vi "rs3 set filter options.vi"(8 "error in (no error)":errorcluster, 10 "Processing Blocks":T2, 11 "Filter settings":T1={"Decimation Scale (1-10)"=3, "Spatial Alpha (0-1)"=0.6, "Spatial Delta (1/32 disp)"=8, "Temporal Alpha (0-1)"=0.4, "Temporal Delta (1/32 disp)"=20, "Persistence (0= none, 8=max)"=0, "spatial holefill radius (0 disable, 5 max) "=0, "spatial iteration (2=default)"=2} {"spatial iteration (2=default)" min=1 max=10; "Decimation Scale (1-10)" min=1 max=10; "Spatial Alpha (0-1)" min=0 max=1 format="%_2g"; "Spatial Delta (1/32 disp)" min=1; "Temporal Alpha (0-1)" min=0 max=1 format="%_2g"; "Temporal Delta (1/32 disp)" min=1; "Persistence (0= none, 8=max)" max=8; "spatial holefill radius (0 disable, 5 max)" max=5}) -> (0 "error out":errorcluster)   [LabVIEW 2017, in "libRealSense3.lvlib"]
doc: "Sets post-processing filter options."
uses:
  libRealSense3.lvlib
panel:
  # "RS3 Set Filter Options"
  # "Spatial Holefill:       \n        0= disabled,\n        1= 2_pixel_radius,\n        2= 4_pixel_radius,\n        3= 8_pixel_radius,\n        4= 6_pixel_radius,\n        5= unlimited_radius"
  # "(C) Intel Corp.,  AGJ"
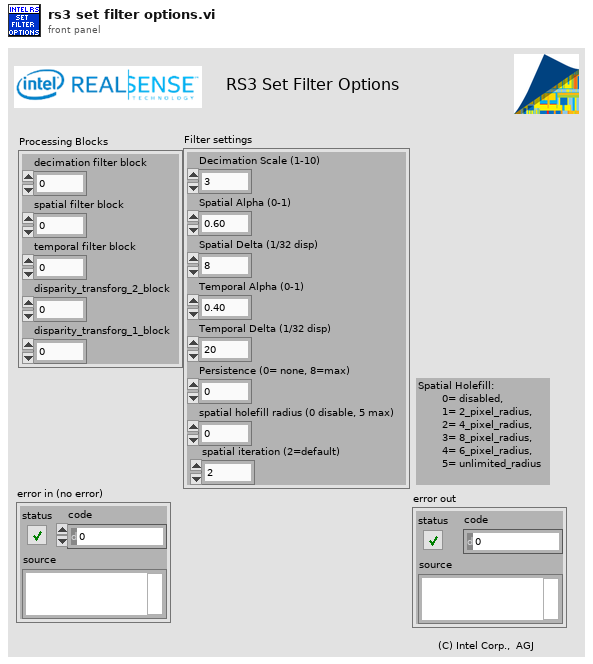
[diagram p1: front panel]
types:
  T1 = cluster{"Decimation Scale (1-10)":u8, "Spatial Alpha (0-1)":sgl, "Spatial Delta (1/32 disp)":u16, "Temporal Alpha (0-1)":sgl, "Temporal Delta (1/32 disp)":u16, "Persistence (0= none, 8=max)":u8, "spatial holefill radius (0 disable, 5 max) ":u8, "spatial iteration (2=default)":u8}
  T2 = cluster{"decimation filter block":u64, "spatial filter block":u64, "temporal filter block":u64, "disparity_transforg_2_block":u64, "disparity_transforg_1_block":u64}
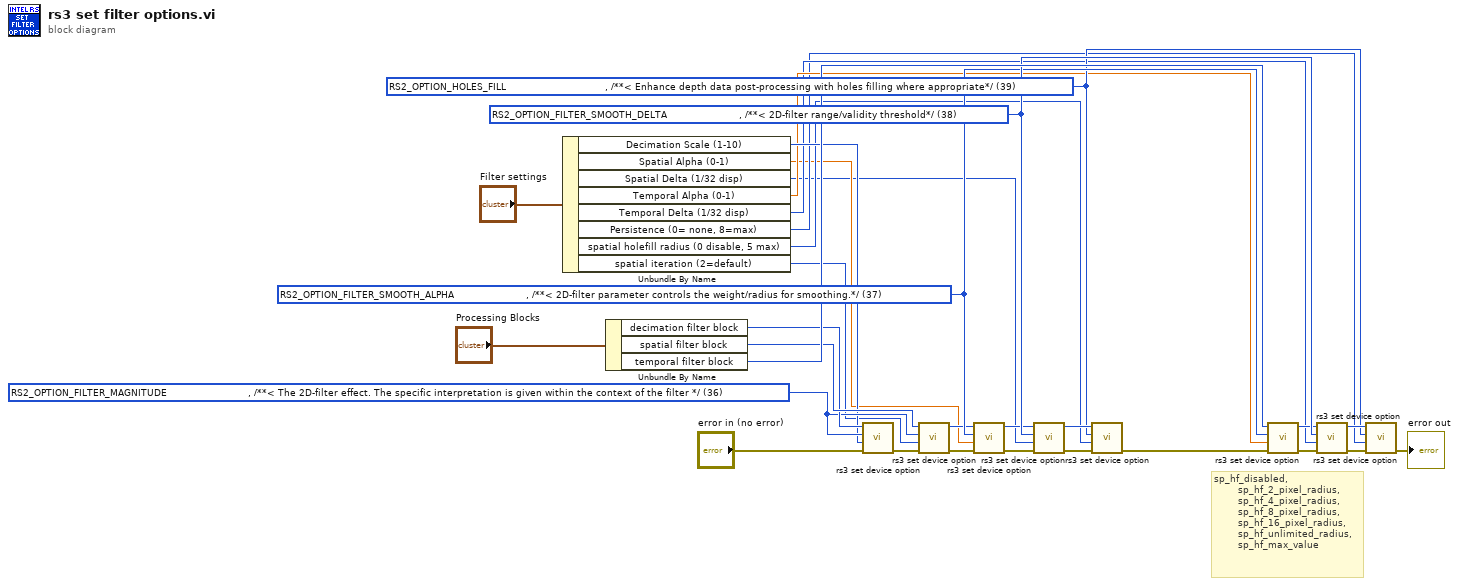
[diagram p0: block diagram]
diagram:
  w9 = u16 39 items=["    RS2_OPTION_BACKLIGHT_COMPENSATION                     , /**< Enable / disable color backlight compensation*/", "    RS2_OPTION_BRIGHTNESS                                 , /**< Color image brightness*/", "    RS2_OPTION_CONTRAST                                   , /**< Color image contrast*/", "    RS2_OPTION_EXPOSURE                                   , /**< Controls exposure time of color camera. Setting any value will disable auto exposure*/", "    RS2_OPTION_GAIN                                       , /**< Color image gain*/", "    RS2_OPTION_GAMMA                                      , /**< Color image gamma setting*/", "    RS2_OPTION_HUE                                        , /**< Color image hue*/", "    RS2_OPTION_SATURATION                                 , /**< Color image saturation setting*/", "    RS2_OPTION_SHARPNESS                                  , /**< Color image sharpness setting*/", "    RS2_OPTION_WHITE_BALANCE                              , /**< Controls white balance of color image. Setting any value will disable auto white balance*/", "    RS2_OPTION_ENABLE_AUTO_EXPOSURE                       , /**< Enable / disable color image auto-exposure*/", "    RS2_OPTION_ENABLE_AUTO_WHITE_BALANCE                  , /**< Enable / disable color image auto-white-balance*/", "    RS2_OPTION_VISUAL_PRESET                              , /**< Provide access to several recommend sets of option presets for the depth camera */", "    RS2_OPTION_LASER_POWER                                , /**< Power of the F200 / SR300 projector, with 0 meaning projector off*/", "    RS2_OPTION_ACCURACY                                   , /**< Set the number of patterns projected per frame. The higher the accuracy value the more patterns projected. Increasing the number of patterns help to achieve better accuracy. Note that this c", "    RS2_OPTION_MOTION_RANGE                               , /**< Motion vs. Range trade-off, with lower values allowing for better motion sensitivity and higher values allowing for better depth range*/", "    RS2_OPTION_FILTER_OPTION                              , /**< Set the filter to apply to each depth frame. Each one of the filter is optimized per the application requirements*/", "    RS2_OPTION_CONFIDENCE_THRESHOLD                       , /**< The confidence level threshold used by the Depth algorithm pipe to set whether a pixel will get a valid range or will be marked with invalid range*/", "    RS2_OPTION_EMITTER_ENABLED                            , /**< Laser Emitter enabled */", "    RS2_OPTION_FRAMES_QUEUE_SIZE                          , /**< Number of frames the user is allowed to keep per stream. Trying to hold-on to more frames will cause frame-drops.*/", "    RS2_OPTION_TOTAL_FRAME_DROPS                          , /**< Total number of detected frame drops from all streams */", "    RS2_OPTION_AUTO_EXPOSURE_MODE                         , /**< Auto-Exposure modes: Static, Anti-Flicker and Hybrid */", "    RS2_OPTION_POWER_LINE_FREQUENCY                       , /**< Power Line Frequency control for anti-flickering Off/50Hz/60Hz/Auto */", "    RS2_OPTION_ASIC_TEMPERATURE                           , /**< Current Asic Temperature */", "    RS2_OPTION_ERROR_POLLING_ENABLED                      , /**< disable error handling */", "    RS2_OPTION_PROJECTOR_TEMPERATURE                      , /**< Current Projector Temperature */", "    RS2_OPTION_OUTPUT_TRIGGER_ENABLED                     , /**< Enable / disable trigger to be outputed from the camera to any external device on every depth frame */", "    RS2_OPTION_MOTION_MODULE_TEMPERATURE                  , /**< Current Motion-Module Temperature */", "    RS2_OPTION_DEPTH_UNITS                                , /**< Number of meters represented by a single depth unit */", "    RS2_OPTION_ENABLE_MOTION_CORRECTION                   , /**< Enable/Disable automatic correction of the motion data */", "    RS2_OPTION_AUTO_EXPOSURE_PRIORITY                     , /**< Allows sensor to dynamically ajust the frame rate depending on lighting conditions */", "    RS2_OPTION_COLOR_SCHEME                               , /**< Color scheme for data visualization */", "    RS2_OPTION_HISTOGRAM_EQUALIZATION_ENABLED             , /**< Perform histogram equalization post-processing on the depth data */", "    RS2_OPTION_MIN_DISTANCE                               , /**< Minimal distance to the target */", "    RS2_OPTION_MAX_DISTANCE                               , /**< Maximum distance to the target */", "    RS2_OPTION_TEXTURE_SOURCE                             , /**< Texture mapping stream unique ID */", "    RS2_OPTION_FILTER_MAGNITUDE                           , /**< The 2D-filter effect. The specific interpretation is given within the context of the filter */", "    RS2_OPTION_FILTER_SMOOTH_ALPHA                        , /**< 2D-filter parameter controls the weight/radius for smoothing.*/", "    RS2_OPTION_FILTER_SMOOTH_DELTA                        , /**< 2D-filter range/validity threshold*/", "    RS2_OPTION_HOLES_FILL                                 , /**< Enhance depth data post-processing with holes filling where appropriate*/", "    RS2_OPTION_STEREO_BASELINE                            , /**< The distance in mm between the first and the second imagers in stereo-based depth cameras*/", "    RS2_OPTION_AUTO_EXPOSURE_CONVERGE_STEP                , /**< Allows dynamically ajust the converge step value of the target exposure in Auto-Exposure algorithm*/", "    RS2_OPTION_COUNT                                        /**< Number of enumeration values. Not a valid input: intended to be used in for-loops. */"] ("RS Option")
  w24 = u16 38 items=["    RS2_OPTION_BACKLIGHT_COMPENSATION                     , /**< Enable / disable color backlight compensation*/", "    RS2_OPTION_BRIGHTNESS                                 , /**< Color image brightness*/", "    RS2_OPTION_CONTRAST                                   , /**< Color image contrast*/", "    RS2_OPTION_EXPOSURE                                   , /**< Controls exposure time of color camera. Setting any value will disable auto exposure*/", "    RS2_OPTION_GAIN                                       , /**< Color image gain*/", "    RS2_OPTION_GAMMA                                      , /**< Color image gamma setting*/", "    RS2_OPTION_HUE                                        , /**< Color image hue*/", "    RS2_OPTION_SATURATION                                 , /**< Color image saturation setting*/", "    RS2_OPTION_SHARPNESS                                  , /**< Color image sharpness setting*/", "    RS2_OPTION_WHITE_BALANCE                              , /**< Controls white balance of color image. Setting any value will disable auto white balance*/", "    RS2_OPTION_ENABLE_AUTO_EXPOSURE                       , /**< Enable / disable color image auto-exposure*/", "    RS2_OPTION_ENABLE_AUTO_WHITE_BALANCE                  , /**< Enable / disable color image auto-white-balance*/", "    RS2_OPTION_VISUAL_PRESET                              , /**< Provide access to several recommend sets of option presets for the depth camera */", "    RS2_OPTION_LASER_POWER                                , /**< Power of the F200 / SR300 projector, with 0 meaning projector off*/", "    RS2_OPTION_ACCURACY                                   , /**< Set the number of patterns projected per frame. The higher the accuracy value the more patterns projected. Increasing the number of patterns help to achieve better accuracy. Note that this c", "    RS2_OPTION_MOTION_RANGE                               , /**< Motion vs. Range trade-off, with lower values allowing for better motion sensitivity and higher values allowing for better depth range*/", "    RS2_OPTION_FILTER_OPTION                              , /**< Set the filter to apply to each depth frame. Each one of the filter is optimized per the application requirements*/", "    RS2_OPTION_CONFIDENCE_THRESHOLD                       , /**< The confidence level threshold used by the Depth algorithm pipe to set whether a pixel will get a valid range or will be marked with invalid range*/", "    RS2_OPTION_EMITTER_ENABLED                            , /**< Laser Emitter enabled */", "    RS2_OPTION_FRAMES_QUEUE_SIZE                          , /**< Number of frames the user is allowed to keep per stream. Trying to hold-on to more frames will cause frame-drops.*/", "    RS2_OPTION_TOTAL_FRAME_DROPS                          , /**< Total number of detected frame drops from all streams */", "    RS2_OPTION_AUTO_EXPOSURE_MODE                         , /**< Auto-Exposure modes: Static, Anti-Flicker and Hybrid */", "    RS2_OPTION_POWER_LINE_FREQUENCY                       , /**< Power Line Frequency control for anti-flickering Off/50Hz/60Hz/Auto */", "    RS2_OPTION_ASIC_TEMPERATURE                           , /**< Current Asic Temperature */", "    RS2_OPTION_ERROR_POLLING_ENABLED                      , /**< disable error handling */", "    RS2_OPTION_PROJECTOR_TEMPERATURE                      , /**< Current Projector Temperature */", "    RS2_OPTION_OUTPUT_TRIGGER_ENABLED                     , /**< Enable / disable trigger to be outputed from the camera to any external device on every depth frame */", "    RS2_OPTION_MOTION_MODULE_TEMPERATURE                  , /**< Current Motion-Module Temperature */", "    RS2_OPTION_DEPTH_UNITS                                , /**< Number of meters represented by a single depth unit */", "    RS2_OPTION_ENABLE_MOTION_CORRECTION                   , /**< Enable/Disable automatic correction of the motion data */", "    RS2_OPTION_AUTO_EXPOSURE_PRIORITY                     , /**< Allows sensor to dynamically ajust the frame rate depending on lighting conditions */", "    RS2_OPTION_COLOR_SCHEME                               , /**< Color scheme for data visualization */", "    RS2_OPTION_HISTOGRAM_EQUALIZATION_ENABLED             , /**< Perform histogram equalization post-processing on the depth data */", "    RS2_OPTION_MIN_DISTANCE                               , /**< Minimal distance to the target */", "    RS2_OPTION_MAX_DISTANCE                               , /**< Maximum distance to the target */", "    RS2_OPTION_TEXTURE_SOURCE                             , /**< Texture mapping stream unique ID */", "    RS2_OPTION_FILTER_MAGNITUDE                           , /**< The 2D-filter effect. The specific interpretation is given within the context of the filter */", "    RS2_OPTION_FILTER_SMOOTH_ALPHA                        , /**< 2D-filter parameter controls the weight/radius for smoothing.*/", "    RS2_OPTION_FILTER_SMOOTH_DELTA                        , /**< 2D-filter range/validity threshold*/", "    RS2_OPTION_HOLES_FILL                                 , /**< Enhance depth data post-processing with holes filling where appropriate*/", "    RS2_OPTION_STEREO_BASELINE                            , /**< The distance in mm between the first and the second imagers in stereo-based depth cameras*/", "    RS2_OPTION_AUTO_EXPOSURE_CONVERGE_STEP                , /**< Allows dynamically ajust the converge step value of the target exposure in Auto-Exposure algorithm*/", "    RS2_OPTION_COUNT                                        /**< Number of enumeration values. Not a valid input: intended to be used in for-loops. */"] ("RS Option")
  w23 = u16 37 items=["    RS2_OPTION_BACKLIGHT_COMPENSATION                     , /**< Enable / disable color backlight compensation*/", "    RS2_OPTION_BRIGHTNESS                                 , /**< Color image brightness*/", "    RS2_OPTION_CONTRAST                                   , /**< Color image contrast*/", "    RS2_OPTION_EXPOSURE                                   , /**< Controls exposure time of color camera. Setting any value will disable auto exposure*/", "    RS2_OPTION_GAIN                                       , /**< Color image gain*/", "    RS2_OPTION_GAMMA                                      , /**< Color image gamma setting*/", "    RS2_OPTION_HUE                                        , /**< Color image hue*/", "    RS2_OPTION_SATURATION                                 , /**< Color image saturation setting*/", "    RS2_OPTION_SHARPNESS                                  , /**< Color image sharpness setting*/", "    RS2_OPTION_WHITE_BALANCE                              , /**< Controls white balance of color image. Setting any value will disable auto white balance*/", "    RS2_OPTION_ENABLE_AUTO_EXPOSURE                       , /**< Enable / disable color image auto-exposure*/", "    RS2_OPTION_ENABLE_AUTO_WHITE_BALANCE                  , /**< Enable / disable color image auto-white-balance*/", "    RS2_OPTION_VISUAL_PRESET                              , /**< Provide access to several recommend sets of option presets for the depth camera */", "    RS2_OPTION_LASER_POWER                                , /**< Power of the F200 / SR300 projector, with 0 meaning projector off*/", "    RS2_OPTION_ACCURACY                                   , /**< Set the number of patterns projected per frame. The higher the accuracy value the more patterns projected. Increasing the number of patterns help to achieve better accuracy. Note that this c", "    RS2_OPTION_MOTION_RANGE                               , /**< Motion vs. Range trade-off, with lower values allowing for better motion sensitivity and higher values allowing for better depth range*/", "    RS2_OPTION_FILTER_OPTION                              , /**< Set the filter to apply to each depth frame. Each one of the filter is optimized per the application requirements*/", "    RS2_OPTION_CONFIDENCE_THRESHOLD                       , /**< The confidence level threshold used by the Depth algorithm pipe to set whether a pixel will get a valid range or will be marked with invalid range*/", "    RS2_OPTION_EMITTER_ENABLED                            , /**< Laser Emitter enabled */", "    RS2_OPTION_FRAMES_QUEUE_SIZE                          , /**< Number of frames the user is allowed to keep per stream. Trying to hold-on to more frames will cause frame-drops.*/", "    RS2_OPTION_TOTAL_FRAME_DROPS                          , /**< Total number of detected frame drops from all streams */", "    RS2_OPTION_AUTO_EXPOSURE_MODE                         , /**< Auto-Exposure modes: Static, Anti-Flicker and Hybrid */", "    RS2_OPTION_POWER_LINE_FREQUENCY                       , /**< Power Line Frequency control for anti-flickering Off/50Hz/60Hz/Auto */", "    RS2_OPTION_ASIC_TEMPERATURE                           , /**< Current Asic Temperature */", "    RS2_OPTION_ERROR_POLLING_ENABLED                      , /**< disable error handling */", "    RS2_OPTION_PROJECTOR_TEMPERATURE                      , /**< Current Projector Temperature */", "    RS2_OPTION_OUTPUT_TRIGGER_ENABLED                     , /**< Enable / disable trigger to be outputed from the camera to any external device on every depth frame */", "    RS2_OPTION_MOTION_MODULE_TEMPERATURE                  , /**< Current Motion-Module Temperature */", "    RS2_OPTION_DEPTH_UNITS                                , /**< Number of meters represented by a single depth unit */", "    RS2_OPTION_ENABLE_MOTION_CORRECTION                   , /**< Enable/Disable automatic correction of the motion data */", "    RS2_OPTION_AUTO_EXPOSURE_PRIORITY                     , /**< Allows sensor to dynamically ajust the frame rate depending on lighting conditions */", "    RS2_OPTION_COLOR_SCHEME                               , /**< Color scheme for data visualization */", "    RS2_OPTION_HISTOGRAM_EQUALIZATION_ENABLED             , /**< Perform histogram equalization post-processing on the depth data */", "    RS2_OPTION_MIN_DISTANCE                               , /**< Minimal distance to the target */", "    RS2_OPTION_MAX_DISTANCE                               , /**< Maximum distance to the target */", "    RS2_OPTION_TEXTURE_SOURCE                             , /**< Texture mapping stream unique ID */", "    RS2_OPTION_FILTER_MAGNITUDE                           , /**< The 2D-filter effect. The specific interpretation is given within the context of the filter */", "    RS2_OPTION_FILTER_SMOOTH_ALPHA                        , /**< 2D-filter parameter controls the weight/radius for smoothing.*/", "    RS2_OPTION_FILTER_SMOOTH_DELTA                        , /**< 2D-filter range/validity threshold*/", "    RS2_OPTION_HOLES_FILL                                 , /**< Enhance depth data post-processing with holes filling where appropriate*/", "    RS2_OPTION_STEREO_BASELINE                            , /**< The distance in mm between the first and the second imagers in stereo-based depth cameras*/", "    RS2_OPTION_AUTO_EXPOSURE_CONVERGE_STEP                , /**< Allows dynamically ajust the converge step value of the target exposure in Auto-Exposure algorithm*/", "    RS2_OPTION_COUNT                                        /**< Number of enumeration values. Not a valid input: intended to be used in for-loops. */"] ("RS Option")
  w16 = u16 36 items=["    RS2_OPTION_BACKLIGHT_COMPENSATION                     , /**< Enable / disable color backlight compensation*/", "    RS2_OPTION_BRIGHTNESS                                 , /**< Color image brightness*/", "    RS2_OPTION_CONTRAST                                   , /**< Color image contrast*/", "    RS2_OPTION_EXPOSURE                                   , /**< Controls exposure time of color camera. Setting any value will disable auto exposure*/", "    RS2_OPTION_GAIN                                       , /**< Color image gain*/", "    RS2_OPTION_GAMMA                                      , /**< Color image gamma setting*/", "    RS2_OPTION_HUE                                        , /**< Color image hue*/", "    RS2_OPTION_SATURATION                                 , /**< Color image saturation setting*/", "    RS2_OPTION_SHARPNESS                                  , /**< Color image sharpness setting*/", "    RS2_OPTION_WHITE_BALANCE                              , /**< Controls white balance of color image. Setting any value will disable auto white balance*/", "    RS2_OPTION_ENABLE_AUTO_EXPOSURE                       , /**< Enable / disable color image auto-exposure*/", "    RS2_OPTION_ENABLE_AUTO_WHITE_BALANCE                  , /**< Enable / disable color image auto-white-balance*/", "    RS2_OPTION_VISUAL_PRESET                              , /**< Provide access to several recommend sets of option presets for the depth camera */", "    RS2_OPTION_LASER_POWER                                , /**< Power of the F200 / SR300 projector, with 0 meaning projector off*/", "    RS2_OPTION_ACCURACY                                   , /**< Set the number of patterns projected per frame. The higher the accuracy value the more patterns projected. Increasing the number of patterns help to achieve better accuracy. Note that this c", "    RS2_OPTION_MOTION_RANGE                               , /**< Motion vs. Range trade-off, with lower values allowing for better motion sensitivity and higher values allowing for better depth range*/", "    RS2_OPTION_FILTER_OPTION                              , /**< Set the filter to apply to each depth frame. Each one of the filter is optimized per the application requirements*/", "    RS2_OPTION_CONFIDENCE_THRESHOLD                       , /**< The confidence level threshold used by the Depth algorithm pipe to set whether a pixel will get a valid range or will be marked with invalid range*/", "    RS2_OPTION_EMITTER_ENABLED                            , /**< Laser Emitter enabled */", "    RS2_OPTION_FRAMES_QUEUE_SIZE                          , /**< Number of frames the user is allowed to keep per stream. Trying to hold-on to more frames will cause frame-drops.*/", "    RS2_OPTION_TOTAL_FRAME_DROPS                          , /**< Total number of detected frame drops from all streams */", "    RS2_OPTION_AUTO_EXPOSURE_MODE                         , /**< Auto-Exposure modes: Static, Anti-Flicker and Hybrid */", "    RS2_OPTION_POWER_LINE_FREQUENCY                       , /**< Power Line Frequency control for anti-flickering Off/50Hz/60Hz/Auto */", "    RS2_OPTION_ASIC_TEMPERATURE                           , /**< Current Asic Temperature */", "    RS2_OPTION_ERROR_POLLING_ENABLED                      , /**< disable error handling */", "    RS2_OPTION_PROJECTOR_TEMPERATURE                      , /**< Current Projector Temperature */", "    RS2_OPTION_OUTPUT_TRIGGER_ENABLED                     , /**< Enable / disable trigger to be outputed from the camera to any external device on every depth frame */", "    RS2_OPTION_MOTION_MODULE_TEMPERATURE                  , /**< Current Motion-Module Temperature */", "    RS2_OPTION_DEPTH_UNITS                                , /**< Number of meters represented by a single depth unit */", "    RS2_OPTION_ENABLE_MOTION_CORRECTION                   , /**< Enable/Disable automatic correction of the motion data */", "    RS2_OPTION_AUTO_EXPOSURE_PRIORITY                     , /**< Allows sensor to dynamically ajust the frame rate depending on lighting conditions */", "    RS2_OPTION_COLOR_SCHEME                               , /**< Color scheme for data visualization */", "    RS2_OPTION_HISTOGRAM_EQUALIZATION_ENABLED             , /**< Perform histogram equalization post-processing on the depth data */", "    RS2_OPTION_MIN_DISTANCE                               , /**< Minimal distance to the target */", "    RS2_OPTION_MAX_DISTANCE                               , /**< Maximum distance to the target */", "    RS2_OPTION_TEXTURE_SOURCE                             , /**< Texture mapping stream unique ID */", "    RS2_OPTION_FILTER_MAGNITUDE                           , /**< The 2D-filter effect. The specific interpretation is given within the context of the filter */", "    RS2_OPTION_FILTER_SMOOTH_ALPHA                        , /**< 2D-filter parameter controls the weight/radius for smoothing.*/", "    RS2_OPTION_FILTER_SMOOTH_DELTA                        , /**< 2D-filter range/validity threshold*/", "    RS2_OPTION_HOLES_FILL                                 , /**< Enhance depth data post-processing with holes filling where appropriate*/", "    RS2_OPTION_STEREO_BASELINE                            , /**< The distance in mm between the first and the second imagers in stereo-based depth cameras*/", "    RS2_OPTION_AUTO_EXPOSURE_CONVERGE_STEP                , /**< Allows dynamically ajust the converge step value of the target exposure in Auto-Exposure algorithm*/", "    RS2_OPTION_COUNT                                        /**< Number of enumeration values. Not a valid input: intended to be used in for-loops. */"] ("RS Option")
  # "sp_hf_disabled,\n        sp_hf_2_pixel_radius,\n        sp_hf_4_pixel_radius,\n        sp_hf_8_pixel_radius,\n        sp_hf_16_pixel_radius,\n        sp_hf_unlimited_radius,\n        sp_hf_max_value"
  n1 = Unbundle By Name("Filter settings") -> ("Decimation Scale (1-10)"=w8:u8, "Spatial Alpha (0-1)"=w2:sgl, "Spatial Delta (1/32 disp)"=w1:u16, "Temporal Alpha (0-1)"=w6:sgl, "Temporal Delta (1/32 disp)"=w5:u16, "Persistence (0= none, 8=max)"=w4:u8, "spatial holefill radius (0 disable, 5 max)"=w3:u8, "spatial iteration (2=default)"=w7:u8)
  n2 = Unbundle By Name("Processing Blocks") -> ("decimation filter block"=w27:u64, "spatial filter block"=w28:u64, "temporal filter block"=w29:u64)
  n3 = call "rs3 set device option.vi"("error in (no error)"="error in (no error)", "value"=w8, "RS Option"=w16, "Sensor in"=w27) -> ("error out"=w15:errorcluster)  [unwired: 5 in, 2 out]
  n4 = call "rs3 set device option.vi"("error in (no error)"=w15, "value"=w7, "RS Option"=w16, "Sensor in"=w28) -> ("error out"=w20:errorcluster, "Sensor out"=w17:u64)  [unwired: 5 in, 1 out]
  n5 = call "rs3 set device option.vi"("error in (no error)"=w20, "value"=w2, "RS Option"=w23, "Sensor in"=w17) -> ("error out"=w18:errorcluster, "Sensor out"=w19:u64)  [unwired: 5 in, 1 out]
  n6 = call "rs3 set device option.vi"("error in (no error)"=w18, "value"=w1, "RS Option"=w24, "Sensor in"=w19) -> ("error out"=w11:errorcluster, "Sensor out"=w12:u64)  [unwired: 5 in, 1 out]
  n7 = call "rs3 set device option.vi"("error in (no error)"=w11, "value"=w3, "RS Option"=w9, "Sensor in"=w12) -> ("error out"=w10:errorcluster)  [unwired: 5 in, 2 out]
  n8 = call "rs3 set device option.vi"("error in (no error)"=w10, "value"=w6, "RS Option"=w23, "Sensor in"=w29) -> ("error out"=w22:errorcluster, "Sensor out"=w21:u64)  [unwired: 5 in, 1 out]
  n9 = call "rs3 set device option.vi"("error in (no error)"=w22, "value"=w5, "RS Option"=w24, "Sensor in"=w21) -> ("error out"=w25:errorcluster, "Sensor out"=w26:u64)  [unwired: 5 in, 1 out]
  n10 = call "rs3 set device option.vi"("error in (no error)"=w25, "value"=w4, "RS Option"=w9, "Sensor in"=w26) -> ("error out"=→"error out":errorcluster)  [unwired: 5 in, 2 out]
